vi "Interpret Driver Controls.vi"() -> ()   [LabVIEW 2018]
uses:
  <vilib>/Rock Robotics/WPI/DriverStation/WPI_DriverStationDerivedRobotMode.ctl
  Robot Global Data.vi
  SubSystems/Controllers/Driver Controller/Driver Controller Global.vi
  SubSystems/Drive Train/Drive Train Global.vi
  SubSystems/Lift/Lift Global.vi
  <vilib>/addons/control/pid/pid.llb/PID (DBL).vi
  SubSystems/Controllers/Manipulator Controlller/Manipulator Controller Global.vi
  SubSystems/HAB Climber/HAB Climber Global.vi
  SubSystems/Hatch Panel Intake/Hatch Panel Intake Global.vi
  SubSystems/Cargo Intake/Cargo Intake Global.vi
  <vilib>/addons/control/pid/NI_PID_pid.lvlib
panel:
  in  "Last Move Deadband":u32=500
  in  "Last Time Auto":u32=1171826
  in  "Camera Tracking":T1={"proportional gain (Kc)"=0.06, "integral time (Ti, min)"=0.0, "derivative time (Td, min)"=0.0}
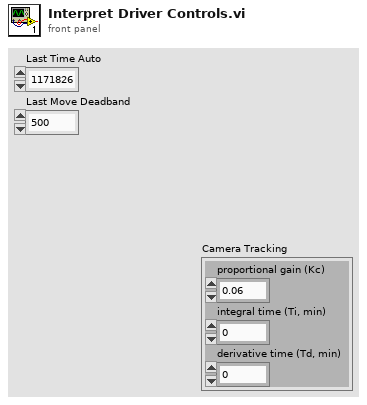
[diagram p1: front panel]
types:
  T1 = cluster{"proportional gain (Kc)":dbl, "integral time (Ti, min)":dbl, "derivative time (Td, min)":dbl}
  T2 = enum16{"Manual", "Hatch Panel Zone 1", "Hatch Panel Zone 2", "Hatch Panel Zone 3", "Cargo Zone 1", "Cargo Zone 2", "Cargo Zone 3", "Cargo Ship Zone"}
  T3 = cluster{"Rollover":dbl, "Yaw":dbl, "Cont Yaw":dbl}
  T4 = typedef "WPI_DriverStationDerivedRobotMode.ctl" = enum16{"Init", "Execute", "Stop"}
  T5 = enum16{"Hatch Panel Zone 1", "Hatch Panel Zone 2", "Hatch Panel Zone 3", "Cargo Zone 1", "Cargo Zone 2", "Cargo Zone 3", "Cargo Ship Zone"}
  T6 = cluster{"offsetAngle H":dbl, "offsetAngle V":dbl, "area":dbl, "skew":dbl, "validTarget":dbl, "latency":dbl}
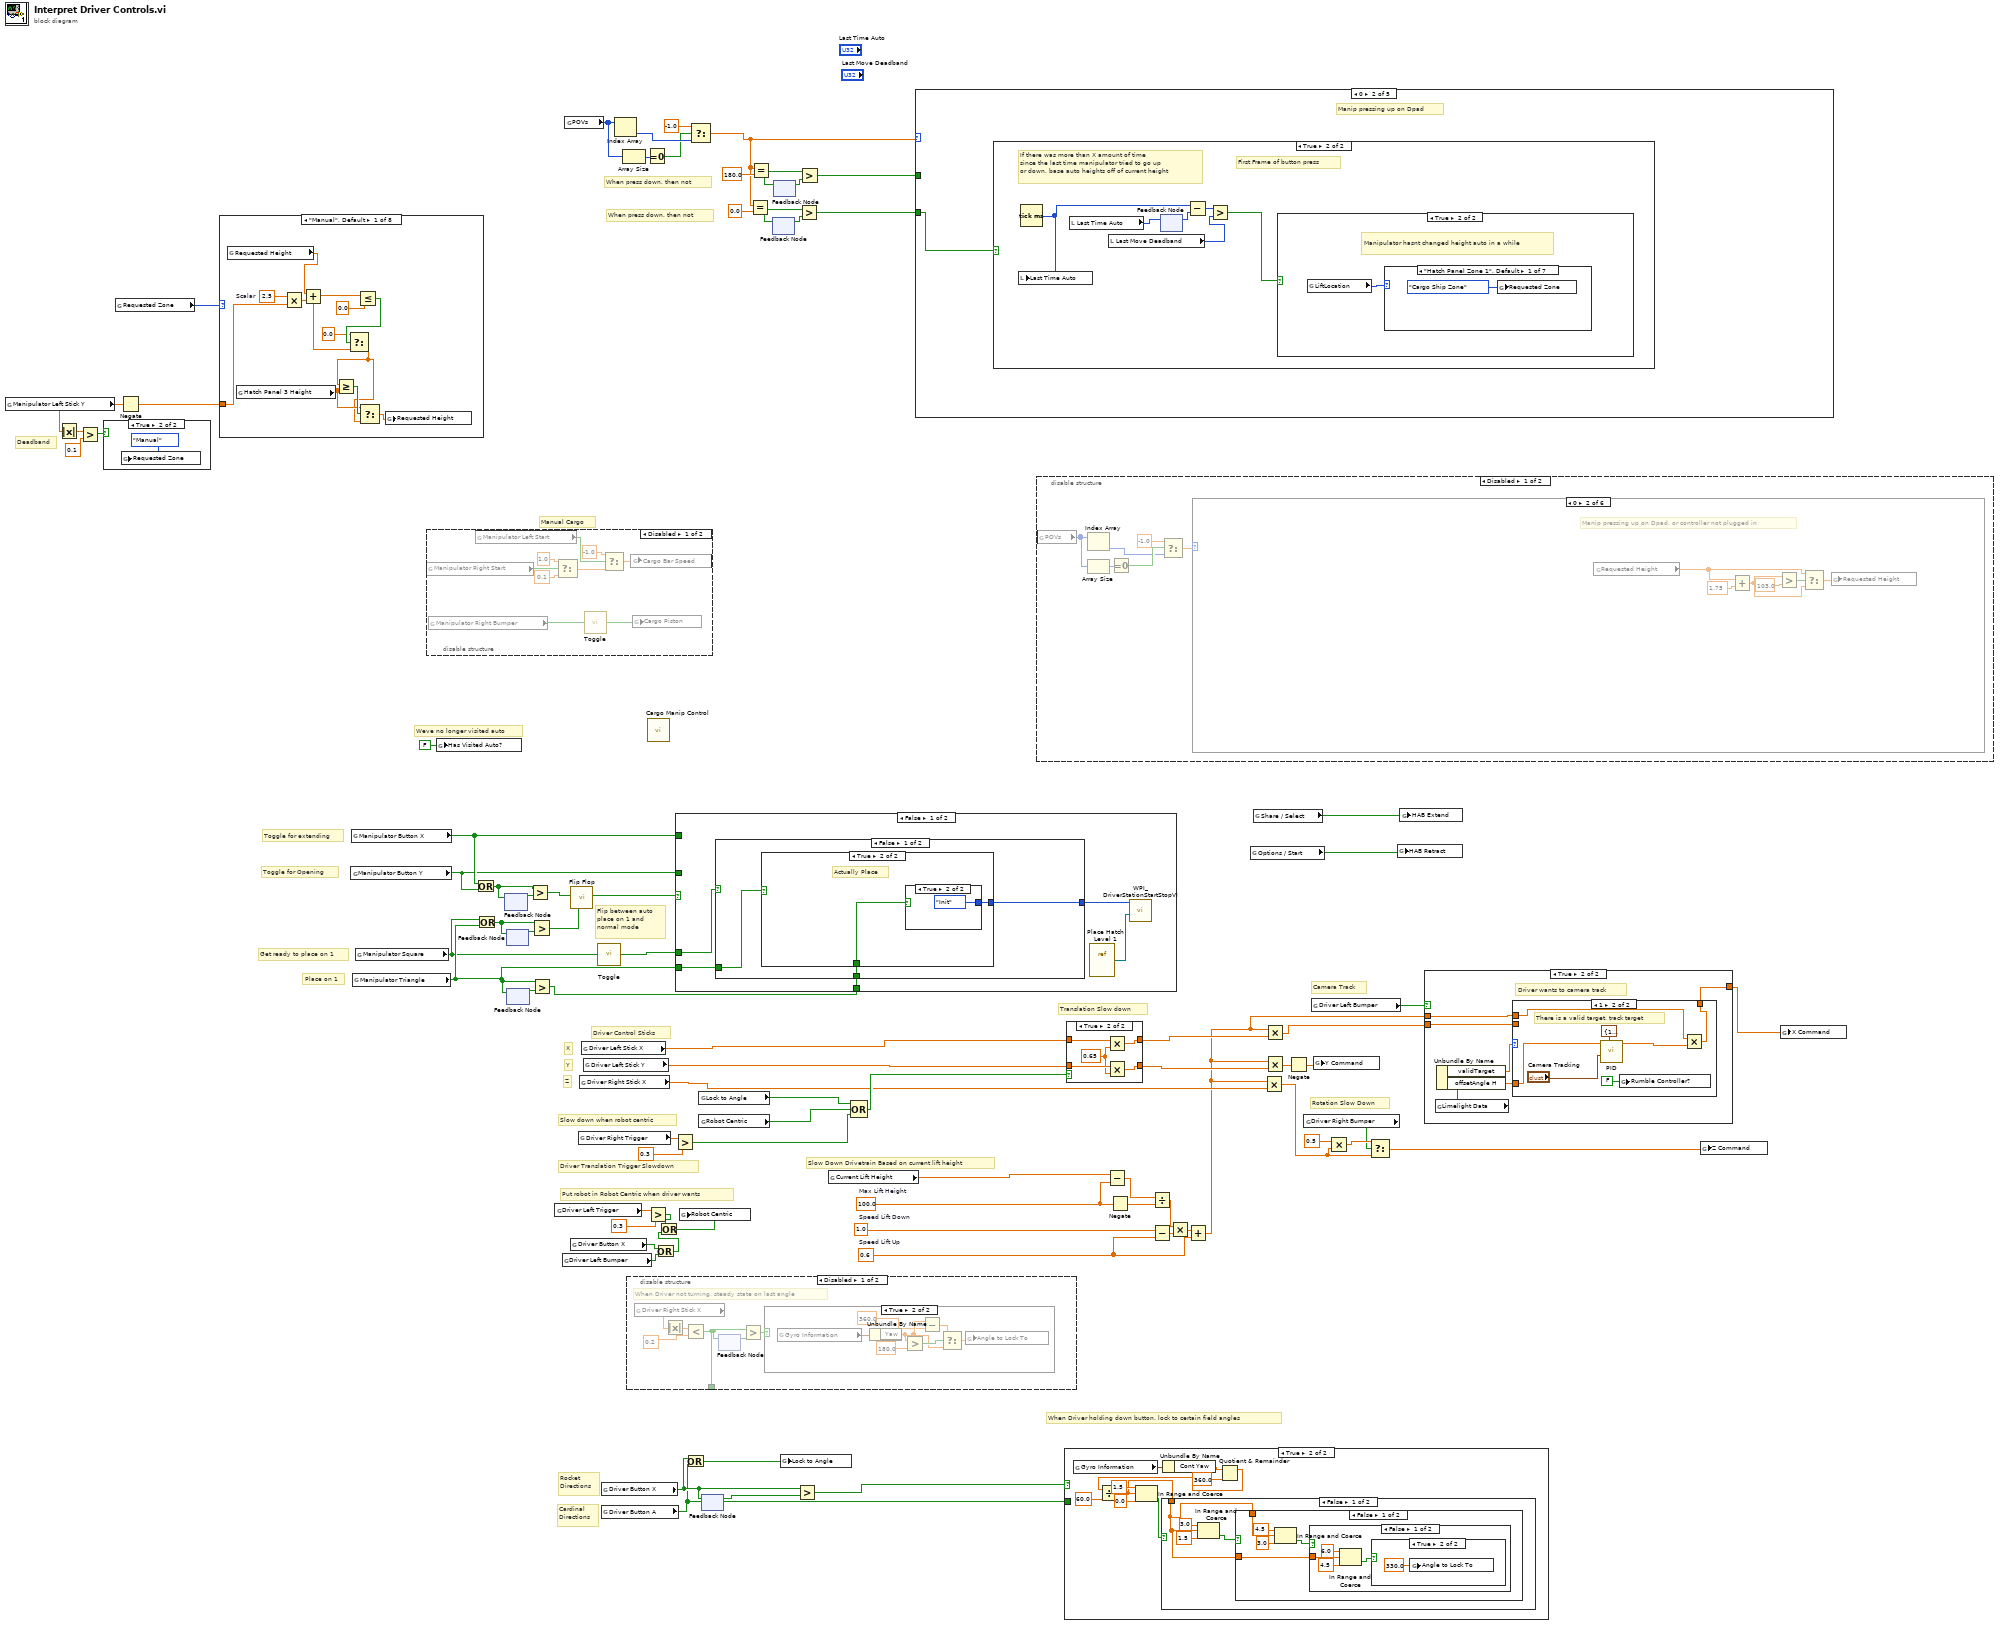
[diagram p0: block diagram]
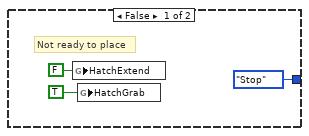
[diagram p2: hidden frame]
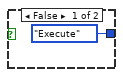
[diagram p3: hidden frame]
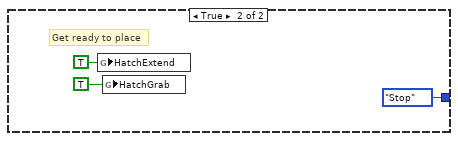
[diagram p4: hidden frame]
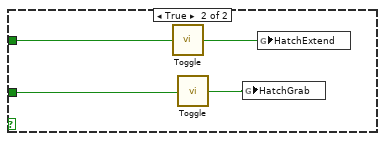
[diagram p5: hidden frame]
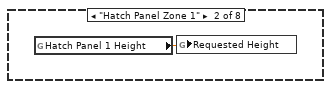
[diagram p7: hidden frame]
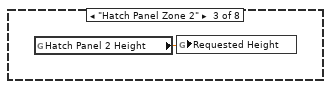
[diagram p8: hidden frame]
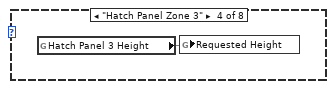
[diagram p9: hidden frame]
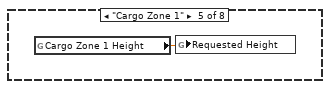
[diagram p10: hidden frame]
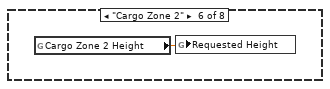
[diagram p11: hidden frame]
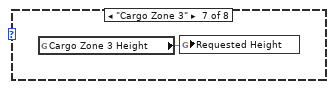
[diagram p12: hidden frame]
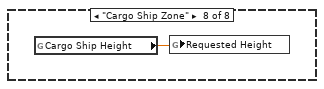
[diagram p13: hidden frame]
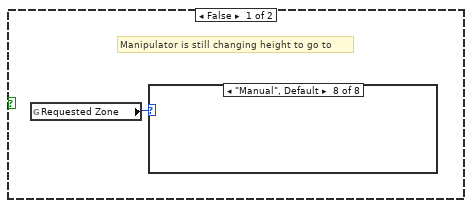
[diagram p16: hidden frame]
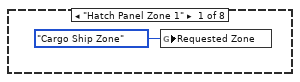
[diagram p17: hidden frame]
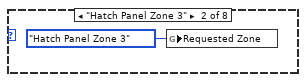
[diagram p18: hidden frame]
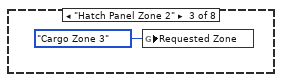
[diagram p19: hidden frame]
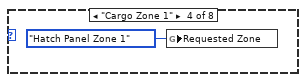
[diagram p20: hidden frame]
diagram:
  w60 = 0.6  # Speed Lift Up
  w64 = 1.0  # Speed Lift Down
  w58 = 100.0  # Max Lift Height
  # "Toggle for Opening"
  # "Toggle for extending"
  # "Place on 1"
  # "Get ready to place on 1"
  # "Flip between auto\nplace on 1 and \nnormal mode"
  # "When press down, then not"
  # "When press down, then not"
  # "Deadband"
  # "Manual Cargo"
  # "Weve no longer visited auto"
  # "Camera Track"
  # "Rotation Slow Down"
  # "Rocket\nDirections"
  # "Cardinal\nDirections"
  # "When Driver holding down button, lock to certain field angles"
  # "Slow Down Drivetrain Based on current lift height"
  # "Put robot in Robot Centric when driver wants"
  # "Slow down when robot centric"
  # "Driver Translation Trigger Slowdown"
  # "Translation Slow down"
  # "Z"
  # "Y"
  # "X"
  # "Driver Control Sticks"
  n1 = global read "Manipulator Controller Global.vi" "Manipulator Left Stick Y"() -> (w27:dbl)
  n2 = Absolute Value(x=w27) -> (abs(x)=w30:dbl)
  n3 = Greater?(x=w30, y=0.1) -> (0:w28:bool)
  n4 = case shown="True" w28 {
    frame False {
    }
    frame True {
      n5 = global write "Lift Global.vi" "Requested Zone"(T2."Manual" ("Requested Zone")) -> ()
    }
  }
  n6 = global read "Lift Global.vi" "Requested Zone"() -> (w31:T2)
  n7 = Negate(x=w27) -> (-x=w26:dbl)
  n8 = case shown="\"Manual\", Default" w31 {
    tunnel: w26 -> [w91 _ _ _ _ _ _ _]
    frame "Manual", Default {
      w90 = 2.5  # Scalar
      n9 = global read "Lift Global.vi" "Requested Height"() -> (w93:dbl)
      n10 = global read "Lift Global.vi" "Hatch Panel 3 Height"() -> (w84:dbl)
      n11 = Multiply(x=w90, y=w91) -> (x*y=w92:dbl)
      n12 = Add(x=w93, y=w92) -> (x+y=w86:dbl)
      n13 = Less Or Equal?(x=w86, y=0.0) -> (x <= y?=w88:bool)
      n14 = Select(t=0.0, s=w88, f=w86) -> (s? t:f=w83:dbl)
      n15 = Greater Or Equal?(x=w83, y=w84) -> (x >= y?=w85:bool)
      n16 = Select(t=w84, s=w85, f=w83) -> (s? t:f=w82:dbl)
      n17 = global write "Lift Global.vi" "Requested Height"(w82) -> ()
    }
    frame "Hatch Panel Zone 1" {
      n18 = global read "Lift Global.vi" "Hatch Panel 1 Height"() -> (w94:dbl)
      n19 = global write "Lift Global.vi" "Requested Height"(w94) -> ()
    }
    frame "Hatch Panel Zone 2" {
      n20 = global read "Lift Global.vi" "Hatch Panel 2 Height"() -> (w95:dbl)
      n21 = global write "Lift Global.vi" "Requested Height"(w95) -> ()
    }
    frame "Hatch Panel Zone 3" {
      n22 = global read "Lift Global.vi" "Hatch Panel 3 Height"() -> (w96:dbl)
      n23 = global write "Lift Global.vi" "Requested Height"(w96) -> ()
    }
    frame "Cargo Zone 1" {
      n24 = global read "Lift Global.vi" "Cargo Zone 1 Height"() -> (w97:dbl)
      n25 = global write "Lift Global.vi" "Requested Height"(w97) -> ()
    }
    frame "Cargo Zone 2" {
      n26 = global read "Lift Global.vi" "Cargo Zone 2 Height"() -> (w98:dbl)
      n27 = global write "Lift Global.vi" "Requested Height"(w98) -> ()
    }
    frame "Cargo Zone 3" {
      n28 = global read "Lift Global.vi" "Cargo Zone 3 Height"() -> (w99:dbl)
      n29 = global write "Lift Global.vi" "Requested Height"(w99) -> ()
    }
    frame "Cargo Ship Zone" {
      n30 = global read "Lift Global.vi" "Cargo Ship Height"() -> (w100:dbl)
      n31 = global write "Lift Global.vi" "Requested Height"(w100) -> ()
    }
  }
  n32 = global read "Manipulator Controller Global.vi" "Manipulator Button Y"() -> (w13:bool)
  n33 = global read "Manipulator Controller Global.vi" "Manipulator Button X"() -> (w14:bool)
  n34 = global read "Manipulator Controller Global.vi" "Manipulator Triangle"() -> (w3:bool)
  n35 = global read "Manipulator Controller Global.vi" "Manipulator Square"() -> (w2:bool)
  n36 = disable-structure shown="Disabled" {
    frame Disabled {
      n37 = global read "Manipulator Controller Global.vi" "Manipulator Right Start"() -> (w106:bool)
      n38 = global read "Manipulator Controller Global.vi" "Manipulator Right Bumper"() -> (w109:bool)
      n39 = global read "Manipulator Controller Global.vi" "Manipulator Left Start"() -> (w105:bool)
      n40 = Select(t=1.0, s=w106, f=0.1) -> (s? t:f=w104:dbl)
      n41 = call "Toggle.vi"("Input"=w109) -> ("Output"=w108:bool)
      n42 = Select(t=-1.0, s=w105, f=w104) -> (s? t:f=w107:dbl)
      n43 = global write "Cargo Intake Global.vi" "Cargo Bar Speed"(w107) -> ()
      n44 = global write "Cargo Intake Global.vi" "Cargo Piston"(w108) -> ()
    }
    frame Enabled {
    }
  }
  n45 = global write "Robot Global Data.vi" "Has Visited Auto?"(FALSE ("Has Visited Auto?")) -> ()
  n46 = Or(x=w14, y=w13) -> (x .or. y?=w11:bool)
  n47 = Or(x=w2, y=w3) -> (x .or. y?=w8:bool)
  n48 = feedback-in #1(w11) -> ()
  n49 = feedback #1() -> (w12:bool)  [unwired: 1 in]
  n50 = feedback #2() -> (w9:bool)  [unwired: 1 in]
  n51 = feedback-in #2(w8) -> ()
  n52 = feedback #3() -> (w5:bool)  [unwired: 1 in]
  n53 = feedback-in #3(w3) -> ()
  n54 = Greater?(x=w11, y=w12) -> (0:w10:bool)
  n55 = Greater?(x=w8, y=w9) -> (0:w7:bool)
  n56 = Greater?(x=w3, y=w5) -> (0:w4:bool)
  n57 = global read "Driver Controller Global.vi" "Driver Left Trigger"() -> (w77:dbl)
  n58 = global read "Driver Controller Global.vi" "Driver Left Bumper"() -> (w43:bool)
  n59 = global read "Manipulator Controller Global.vi" "POVs"() -> (w35:i16[])
  n60 = call "Flip Flop.vi"("Line 2"=w7, "Line 1"=w10) -> ("Switch"=w6:bool)  [unwired: 9 in]
  n61 = global read "Driver Controller Global.vi" "Driver Button X"() -> (w44:bool)
  n62 = global read "Driver Controller Global.vi" "Driver Right Trigger"() -> (w80:dbl)
  n63 = global read "Driver Controller Global.vi" "Driver Right Stick X"() -> (w36:dbl)
  n64 = global read "Driver Controller Global.vi" "Driver Left Stick X"() -> (w37:dbl)
  n65 = global read "Driver Controller Global.vi" "Driver Left Stick Y"() -> (w67:dbl)
  n66 = call "Toggle.vi"("Input"=w2) -> ("Output"=w1:bool)
  n67 = global read "Driver Controller Global.vi" "Driver Button X"() -> (w56:bool)
  n68 = global read "Driver Controller Global.vi" "Driver Button A"() -> (w54:bool)
  n69 = Index Array(array=w35) -> (element=w32:i16)  [unwired: 1 in]
  n70 = Array Size(array=w35) -> (size(s)=w34:i32)
  n71 = disable-structure shown="Disabled" {
    disable-tunnel: [w110 _] -> _
    frame Disabled {
      # "When Driver not turning, steady state on last angle"
      n72 = global read "Driver Controller Global.vi" "Driver Right Stick X"() -> (w111:dbl)
      n73 = Absolute Value(x=w111) -> (abs(x)=w115:dbl)
      n74 = Less?(x=w115, y=0.2) -> (x < y?=w110:bool)
      n75 = feedback #4() -> (w113:bool)  [unwired: 1 in]
      n76 = feedback-in #4(w110) -> ()
      n77 = Greater?(x=w110, y=w113) -> (0:w112:bool)
      n78 = case shown="True" w112 {
        frame False {
        }
        frame True {
          n79 = global read "Drive Train Global.vi" "Gyro Information"() -> (w122:T3)
          n80 = Unbundle By Name(w122) -> ("Yaw"=w119:dbl)
          n81 = Greater?(x=w119, y=180.0) -> (0:w120:bool)
          n82 = Subtract(x=w119, y=360.0) -> (x-y=w117:dbl)
          n83 = Select(t=w117, s=w120, f=w119) -> (s? t:f=w116:dbl)
          n84 = global write "Drive Train Global.vi" "Angle to Lock To"(w116) -> ()
        }
      }
    }
    frame Enabled {
    }
  }
  n85 = Equal To 0?(x=w34) -> (x = 0?=w25:bool)
  n86 = call "Cargo Manip Control.vi"() -> ()  [unwired: 12 in]
  n87 = Greater?(x=w77, y=0.3) -> (0:w52:bool)
  n88 = Or(x=w44, y=w43) -> (x .or. y?=w45:bool)
  n89 = Or(x=w52, y=w45) -> (x .or. y?=w50:bool)
  n90 = Greater?(x=w80, y=0.3) -> (0:w72:bool)
  n91 = case shown="False" w6 {
    tunnel: w13 -> [_ w144]
    tunnel: w14 -> [_ w142]
    tunnel: w1 -> [w127 _]
    tunnel: w4 -> [w124 _]
    tunnel: w3 -> [w123 _]
    frame False {
      n92 = case shown="False" w127 {
        tunnel: [w130 WPI_DriverStationDerivedRobotMode."Stop" ("Call Context")] -> w125
        tunnel: w124 -> [w129 _]
        tunnel: w123 -> [w128 _]
        frame False {
          n93 = case shown="True" w128 {
            tunnel: [WPI_DriverStationDerivedRobotMode."Stop" ("Call Context") w135] -> w130
            tunnel: w129 -> [_ w134]
            frame False {
              # "Not ready to place"
              n94 = global write "Hatch Panel Intake Global.vi" "HatchExtend"(FALSE ("HatchExtend")) -> ()
              n95 = global write "Hatch Panel Intake Global.vi" "HatchGrab"(TRUE ("HatchExtend")) -> ()
            }
            frame True {
              # "Actually Place"
              n96 = case shown="True" w134 {
                tunnel: [WPI_DriverStationDerivedRobotMode."Execute" ("Call Context") WPI_DriverStationDerivedRobotMode."Init" ("Call Context")] -> w135
                frame False {
                }
                frame True {
                }
              }
            }
          }
        }
        frame True {
          # "Get ready to place"
          n97 = global write "Hatch Panel Intake Global.vi" "HatchExtend"(TRUE ("HatchExtend")) -> ()
          n98 = global write "Hatch Panel Intake Global.vi" "HatchGrab"(TRUE ("HatchExtend")) -> ()
        }
      }
      n99 = vi-ref "Place Hatch Level 1.vi"() -> (w126:refnum<vi>)
      n100 = call <vilib>:"WPI_DriverStationStartStopVI.vi"("VI in"=w126, "Call Context"=w125) -> ()  [unwired: 10 in]
    }
    frame True {
      n101 = call "Toggle.vi"("Input"=w142) -> ("Output"=w143:bool)
      n102 = call "Toggle.vi"("Input"=w144) -> ("Output"=w141:bool)
      n103 = global write "Hatch Panel Intake Global.vi" "HatchGrab"(w141) -> ()
      n104 = global write "Hatch Panel Intake Global.vi" "HatchExtend"(w143) -> ()
    }
  }
  n105 = global write "Drive Train Global.vi" "Robot Centric"(w50) -> ()
  n106 = Or(x=w56, y=w54) -> (x .or. y?=w53:bool)
  n107 = Select(t=-1.0, s=w25, f=w32) -> (s? t:f=w17:dbl)
  n108 = global read "Drive Train Global.vi" "Lock to Angle"() -> (w51:bool)
  n109 = global read "Drive Train Global.vi" "Robot Centric"() -> (w71:bool)
  n110 = feedback #5() -> (w57:bool)  [unwired: 1 in]
  n111 = feedback-in #5(w56) -> ()
  n112 = Equal?(x=w17, y=0.0) -> (x = y?=w20:bool)
  n113 = Equal?(x=w17, y=180.0) -> (x = y?=w22:bool)
  n114 = feedback #6() -> (w19:bool)  [unwired: 1 in]
  n115 = feedback-in #6(w20) -> ()
  n116 = feedback-in #7(w22) -> ()
  n117 = feedback #7() -> (w23:bool)  [unwired: 1 in]
  n118 = global write "Drive Train Global.vi" "Lock to Angle"(w53) -> ()
  n119 = Greater?(x=w56, y=w57) -> (0:w55:bool)
  n120 = Greater?(x=w20, y=w19) -> (0:w16:bool)
  n121 = Greater?(x=w22, y=w23) -> (0:w21:bool)
  n122 = global read "Lift Global.vi" "Current Lift Height"() -> (w66:dbl)
  n123 = Compound Arithmetic op=OR(w51, w71, w72) -> (w70:bool)
  n124 = case shown="0" w17 {
    tunnel: w21 -> [_ _ w168 _ _]
    tunnel: w16 -> [_ w145 _ _ _]
    frame -1, Default {
      # "Nothing on the D-Pad is pressed!"
    }
    frame 0 {
      # "Manip pressing up on Dpad"
      n125 = case shown="True" w145 {
        frame False {
          # "Still pressing button, do nothing"
        }
        frame True {
          # "First Frame of button press"
          # "If there was more than X amount of time\nsince the last time manipulator tried to go up\nor down, base auto heights off of current height"
          n126 = Tick Count (ms)() -> (millisecond timer value=w148:u32)
          n127 = local write "Last Time Auto"(w148) -> ()
          n128 = local read "Last Time Auto"() -> (w147:u32)
          n129 = local read "Last Move Deadband"() -> (w149:u32)
          n130 = feedback #8() -> (w146:u32)  [unwired: 1 in]
          n131 = feedback-in #8(w147) -> ()
          n132 = Subtract(x=w148, y=w146) -> (x-y=w151:u32)
          n133 = Greater?(x=w151, y=w149) -> (0:w150:bool)
          n134 = case shown="True" w150 {
            frame False {
              # "Manipulator is still changing height to go to"
              n135 = global read "Lift Global.vi" "Requested Zone"() -> (w152:T2)
              n136 = case shown="\"Manual\", Default" w152 {
                frame "Hatch Panel Zone 1" {
                  n137 = global write "Lift Global.vi" "Requested Zone"(T2."Cargo Ship Zone" ("Requested Zone")) -> ()
                }
                frame "Hatch Panel Zone 3" {
                  n138 = global write "Lift Global.vi" "Requested Zone"(T2."Hatch Panel Zone 3" ("Requested Zone")) -> ()
                }
                frame "Hatch Panel Zone 2" {
                  n139 = global write "Lift Global.vi" "Requested Zone"(T2."Cargo Zone 3" ("Requested Zone")) -> ()
                }
                frame "Cargo Zone 1" {
                  n140 = global write "Lift Global.vi" "Requested Zone"(T2."Hatch Panel Zone 1" ("Requested Zone")) -> ()
                }
                frame "Cargo Zone 2" {
                  n141 = global write "Lift Global.vi" "Requested Zone"(T2."Hatch Panel Zone 2" ("Requested Zone")) -> ()
                }
                frame "Cargo Zone 3" {
                  n142 = global write "Lift Global.vi" "Requested Zone"(T2."Hatch Panel Zone 3" ("Requested Zone")) -> ()
                }
                frame "Cargo Ship Zone" {
                  n143 = global write "Lift Global.vi" "Requested Zone"(T2."Cargo Zone 2" ("Requested Zone")) -> ()
                }
                frame "Manual", Default {
                }
              }
            }
            frame True {
              # "Manipulator hasnt changed height auto in a while"
              n144 = global read "Lift Global.vi" "LiftLocation"() -> (w160:T5)
              n145 = case shown="\"Hatch Panel Zone 1\", Default" w160 {
                frame "Hatch Panel Zone 1", Default {
                  n146 = global write "Lift Global.vi" "Requested Zone"(T2."Cargo Ship Zone" ("Requested Zone")) -> ()
                }
                frame "Hatch Panel Zone 3" {
                  n147 = global write "Lift Global.vi" "Requested Zone"(T2."Hatch Panel Zone 3" ("Requested Zone")) -> ()
                }
                frame "Hatch Panel Zone 2" {
                  n148 = global write "Lift Global.vi" "Requested Zone"(T2."Cargo Zone 3" ("Requested Zone")) -> ()
                }
                frame "Cargo Zone 1" {
                  n149 = global write "Lift Global.vi" "Requested Zone"(T2."Hatch Panel Zone 1" ("Requested Zone")) -> ()
                }
                frame "Cargo Zone 2" {
                  n150 = global write "Lift Global.vi" "Requested Zone"(T2."Hatch Panel Zone 2" ("Requested Zone")) -> ()
                }
                frame "Cargo Zone 3" {
                  n151 = global write "Lift Global.vi" "Requested Zone"(T2."Hatch Panel Zone 3" ("Requested Zone")) -> ()
                }
                frame "Cargo Ship Zone" {
                  n152 = global write "Lift Global.vi" "Requested Zone"(T2."Cargo Zone 2" ("Requested Zone")) -> ()
                }
              }
            }
          }
        }
      }
    }
    frame 180 {
      # "Manip pressing down on Dpad"
      n153 = case shown="True" w168 {
        frame False {
          # "Still pressing button, do nothing"
        }
        frame True {
          # "First frame of button press"
          # "If there was more than X amount of time\nsince the last time manipulator tried to go up\nor down, base auto heights off of current height"
          n154 = Tick Count (ms)() -> (millisecond timer value=w173:u32)
          n155 = local write "Last Time Auto"(w173) -> ()
          n156 = local read "Last Time Auto"() -> (w170:u32)
          n157 = local read "Last Move Deadband"() -> (w172:u32)
          n158 = feedback #9() -> (w169:u32)  [unwired: 1 in]
          n159 = feedback-in #9(w170) -> ()
          n160 = Subtract(x=w173, y=w169) -> (x-y=w174:u32)
          n161 = Greater?(x=w174, y=w172) -> (0:w171:bool)
          n162 = case shown="False" w171 {
            frame False {
              # "Manipulator is still changing height to go to"
              n163 = global read "Lift Global.vi" "Requested Zone"() -> (w175:T2)
              n164 = case shown="\"Cargo Ship Zone\"" w175 {
                frame "Hatch Panel Zone 1" {
                  n165 = global write "Lift Global.vi" "Requested Zone"(T2."Cargo Zone 1" ("Requested Zone")) -> ()
                }
                frame "Hatch Panel Zone 3" {
                  n166 = global write "Lift Global.vi" "Requested Zone"(T2."Cargo Zone 3" ("Requested Zone")) -> ()
                }
                frame "Hatch Panel Zone 2" {
                  n167 = global write "Lift Global.vi" "Requested Zone"(T2."Cargo Zone 2" ("Requested Zone")) -> ()
                }
                frame "Cargo Zone 1" {
                  n168 = global write "Lift Global.vi" "Requested Zone"(T2."Cargo Zone 1" ("Requested Zone")) -> ()
                }
                frame "Cargo Zone 2" {
                  n169 = global write "Lift Global.vi" "Requested Zone"(T2."Cargo Ship Zone" ("Requested Zone")) -> ()
                }
                frame "Cargo Zone 3" {
                  n170 = global write "Lift Global.vi" "Requested Zone"(T2."Hatch Panel Zone 2" ("Requested Zone")) -> ()
                }
                frame "Cargo Ship Zone" {
                  n171 = global write "Lift Global.vi" "Requested Zone"(T2."Hatch Panel Zone 1" ("Requested Zone")) -> ()
                }
                frame "Manual", Default {
                }
              }
            }
            frame True {
              # "Manipulator hasnt changed height auto in a while"
              n172 = global read "Lift Global.vi" "LiftLocation"() -> (w183:T5)
              n173 = case shown="\"Hatch Panel Zone 1\", Default" w183 {
                frame "Hatch Panel Zone 1", Default {
                  n174 = global write "Lift Global.vi" "Requested Zone"(T2."Cargo Zone 1" ("Requested Zone")) -> ()
                }
                frame "Hatch Panel Zone 3" {
                  n175 = global write "Lift Global.vi" "Requested Zone"(T2."Cargo Zone 3" ("Requested Zone")) -> ()
                }
                frame "Hatch Panel Zone 2" {
                  n176 = global write "Lift Global.vi" "Requested Zone"(T2."Cargo Zone 2" ("Requested Zone")) -> ()
                }
                frame "Cargo Zone 1" {
                  n177 = global write "Lift Global.vi" "Requested Zone"(T2."Cargo Zone 1" ("Requested Zone")) -> ()
                }
                frame "Cargo Zone 2" {
                  n178 = global write "Lift Global.vi" "Requested Zone"(T2."Cargo Ship Zone" ("Requested Zone")) -> ()
                }
                frame "Cargo Zone 3" {
                  n179 = global write "Lift Global.vi" "Requested Zone"(T2."Hatch Panel Zone 2" ("Requested Zone")) -> ()
                }
                frame "Cargo Ship Zone" {
                  n180 = global write "Lift Global.vi" "Requested Zone"(T2."Hatch Panel Zone 1" ("Requested Zone")) -> ()
                }
              }
            }
          }
        }
      }
    }
    frame 90 {
      # "Go to Cargo in Cargo Ship Height"
      # "Right on D-Pad"
      n181 = global write "Lift Global.vi" "Requested Zone"(T2."Cargo Ship Zone" ("Requested Zone")) -> ()
    }
    frame 270 {
      # "Go to Hatch Level 1 Height"
      # "Left on D-Pad"
      n182 = global write "Lift Global.vi" "Requested Zone"(T2."Hatch Panel Zone 1" ("Requested Zone")) -> ()
    }
  }
  n183 = disable-structure shown="Disabled" {
    frame Disabled {
      n184 = global read "Manipulator Controller Global.vi" "POVs"() -> (w198:i16[])
      n185 = Index Array(array=w198) -> (element=w193:i16)  [unwired: 1 in]
      n186 = Array Size(array=w198) -> (size(s)=w197:i32)
      n187 = Equal To 0?(x=w197) -> (x = 0?=w195:bool)
      n188 = Select(t=-1.0, s=w195, f=w193) -> (s? t:f=w196:dbl)
      n189 = case shown="0" w196 {
        frame -1 {
          # "If the value changed (manip pressed button)\nchange set lift height to match"
          # "When button goes from\nnot pressed to pressed"
          n190 = global read "Manipulator Controller Global.vi" "Manipulator Square"() -> (w204:bool)
          n191 = feedback #10() -> (w205:bool)  [unwired: 1 in]
          n192 = feedback-in #10(w204) -> ()
          n193 = Greater?(x=w204, y=w205) -> (0:w201:bool)
          n194 = feedback #11() -> (w199:dbl)  [unwired: 1 in]
          n195 = feedback #12() -> (w203:dbl)  [unwired: 1 in]
          n196 = case shown="False" w201 {
            tunnel: [w215 w230] -> w200
            tunnel: w203 -> [w216 w229]
            frame False {
              # "When button goes from\nnot pressed to pressed"
              n197 = global read "Manipulator Controller Global.vi" "Manipulator Triangle"() -> (w218:bool)
              n198 = feedback #13() -> (w217:bool)  [unwired: 1 in]
              n199 = feedback-in #13(w218) -> ()
              n200 = Greater?(x=w218, y=w217) -> (0:w214:bool)
              n201 = case shown="True" w214 {
                tunnel: w216 -> [w219 w221]
                tunnel: [w219 w223] -> w215
                frame False {
                }
                frame True {
                  # "If counter smaller than 5\nadd 1"
                  n202 = Less?(x=w221, y=5.0) -> (x < y?=w220:bool)
                  n203 = case shown="True" w220 {
                    tunnel: [w224 w226] -> w223
                    tunnel: w221 -> [w224 w225]
                    frame False {
                    }
                    frame True {
                      n204 = Increment(x=w225) -> (x+1=w226:dbl)
                    }
                  }
                }
              }
            }
            frame True {
              # "If counter bigger than 0\nsubtract 1"
              n205 = Greater?(x=w229, y=0.0) -> (0:w228:bool)
              n206 = case shown="False" w228 {
                tunnel: [0.0 ("y") w233] -> w230
                tunnel: w229 -> [_ w232]
                frame False {
                }
                frame True {
                  n207 = Decrement(x=w232) -> (x-1=w233:dbl)
                }
              }
            }
          }
          n208 = feedback-in #11(w200) -> ()
          n209 = Not Equal?(x=w200, y=w199) -> (x != y?=w202:bool)
          n210 = case shown="True" w202 {
            tunnel: w200 -> [_ w206]
            frame False {
              # "Manipulator didnt request change"
            }
            frame True {
              # "Set height request to new value"
              n211 = case shown="0, Default" w206 {
                tunnel: [w208 w209 w210 w211 w212 w213] -> w207
                frame 0, Default {
                  n212 = global read "Lift Global.vi" "Cargo Zone 1 Height"() -> (w208:dbl)
                }
                frame 1 {
                  n213 = global read "Lift Global.vi" "Hatch Panel 1 Height"() -> (w209:dbl)
                }
                frame 2 {
                  n214 = global read "Lift Global.vi" "Cargo Zone 2 Height"() -> (w210:dbl)
                }
                frame 3 {
                  n215 = global read "Lift Global.vi" "Hatch Panel 2 Height"() -> (w211:dbl)
                }
                frame 4 {
                  n216 = global read "Lift Global.vi" "Cargo Zone 3 Height"() -> (w212:dbl)
                }
                frame 5 {
                  n217 = global read "Lift Global.vi" "Hatch Panel 3 Height"() -> (w213:dbl)
                }
              }
              n218 = global write "Lift Global.vi" "Requested Height"(w207) -> ()
            }
          }
          n219 = global write "Lift Global.vi" "Lift Auto Position"(w200) -> ()
          n220 = feedback-in #12(w200) -> ()
        }
        frame 0 {
          # "Manip pressing up on Dpad, or controller not plugged in"
          n221 = global read "Lift Global.vi" "Requested Height"() -> (w235:dbl)
          n222 = Add(x=w235, y=1.75) -> (x+y=w234:dbl)
          n223 = Greater?(x=w234, y=103.0) -> (0:w236:bool)
          n224 = Select(t=w235, s=w236, f=w234) -> (s? t:f=w237:dbl)
          n225 = global write "Lift Global.vi" "Requested Height"(w237) -> ()
        }
        frame 180 {
          # "Manip pressing down on Dpad"
          n226 = global read "Lift Global.vi" "Requested Height"() -> (w240:dbl)
          n227 = Add(x=w240, y=-1.0) -> (x+y=w242:dbl)
          n228 = Less?(x=w242, y=0.0) -> (x < y?=w243:bool)
          n229 = Select(t=w240, s=w243, f=w242) -> (s? t:f=w241:dbl)
          n230 = global write "Lift Global.vi" "Requested Height"(w241) -> ()
        }
        frame 90 {
          # "Go to Cargo in Cargo Ship Height"
          # "Right on D-Pad"
          n231 = global read "Lift Global.vi" "Cargo Ship Height"() -> (w246:dbl)
          n232 = global write "Lift Global.vi" "Requested Height"(w246) -> ()
        }
        frame 270 {
          # "Go to Hatch Level 1 Height"
          # "Left on D-Pad"
          n233 = global read "Lift Global.vi" "Hatch Panel 1 Height"() -> (w247:dbl)
          n234 = global write "Lift Global.vi" "Requested Height"(w247) -> ()
        }
        frame -100, Default {
        }
      }
    }
    frame Enabled {
    }
  }
  n235 = case shown="True" w55 {
    tunnel: w54 -> [w249 _]
    frame False {
      n236 = feedback #14() -> (w250:bool)  [unwired: 1 in]
      n237 = feedback-in #14(w249) -> ()
      n238 = Greater?(x=w249, y=w250) -> (0:w248:bool)
      n239 = case shown="True" w248 {
        frame False {
        }
        frame True {
          n240 = global read "Drive Train Global.vi" "Gyro Information"() -> (w257:T3)
          n241 = Unbundle By Name(w257) -> ("Yaw"=w254:dbl)
          n242 = Add(x=w254, y=180.0) -> (x+y=w253:dbl)
          n243 = Divide(x=w253, y=90.0) -> (x/y=w255:dbl)
          n244 = Round To Nearest(number=w255) -> (nearest integer value=w251:dbl)
          n245 = case shown="1" w251 {
            frame 0, Default {
              n246 = global write "Drive Train Global.vi" "Angle to Lock To"(180.0 ("Angle to Lock To")) -> ()
            }
            frame 1 {
              n247 = global write "Drive Train Global.vi" "Angle to Lock To"(270.0 ("Angle to Lock To")) -> ()
            }
            frame 2 {
              n248 = global write "Drive Train Global.vi" "Angle to Lock To"(0.0 ("Angle to Lock To")) -> ()
            }
            frame 3 {
              n249 = global write "Drive Train Global.vi" "Angle to Lock To"(90.0 ("Angle to Lock To")) -> ()
            }
            frame 4 {
              n250 = global write "Drive Train Global.vi" "Angle to Lock To"(180.0 ("Angle to Lock To")) -> ()
            }
          }
        }
      }
    }
    frame True {
      n251 = global read "Drive Train Global.vi" "Gyro Information"() -> (w271:T3)
      n252 = Unbundle By Name(w271) -> ("Cont Yaw"=w269:dbl)
      n253 = Quotient & Remainder(x=w269, y=360.0) -> (x-y*floor(x/y)=w267:dbl)  [unwired: 1 out]
      n254 = Divide(x=w267, y=60.0) -> (x/y=w263:dbl)
      n255 = In Range and Coerce(upper limit=1.5, x=w263, lower limit=0.0) -> (In Range?=w264:bool)  [unwired: 1 out]
      n256 = case shown="False" w264 {
        tunnel: w263 -> [w272 _]
        frame False {
          n257 = In Range and Coerce(upper limit=3.0, x=w272, lower limit=1.5) -> (In Range?=w273:bool)  [unwired: 1 out]
          n258 = case shown="False" w273 {
            tunnel: w272 -> [w278 _]
            tunnel: w272 -> [w276 _]
            frame False {
              n259 = In Range and Coerce(upper limit=4.5, x=w278, lower limit=3.0) -> (In Range?=w277:bool)  [unwired: 1 out]
              n260 = case shown="False" w277 {
                tunnel: w276 -> [w282 _]
                frame False {
                  n261 = In Range and Coerce(upper limit=6.0, x=w282, lower limit=4.5) -> (In Range?=w281:bool)  [unwired: 1 out]
                  n262 = case shown="True" w281 {
                    frame False {
                    }
                    frame True {
                      n263 = global write "Drive Train Global.vi" "Angle to Lock To"(330.0 ("Angle to Lock To")) -> ()
                    }
                  }
                }
                frame True {
                  n264 = global write "Drive Train Global.vi" "Angle to Lock To"(210.0 ("Angle to Lock To")) -> ()
                }
              }
            }
            frame True {
              n265 = global write "Drive Train Global.vi" "Angle to Lock To"(150.0 ("Angle to Lock To")) -> ()
            }
          }
        }
        frame True {
          n266 = global write "Drive Train Global.vi" "Angle to Lock To"(30.0 ("Angle to Lock To")) -> ()
        }
      }
    }
  }
  n267 = case shown="True" w70 {
    tunnel: w67 -> [w290 w295]
    tunnel: [w290 w294] -> w69
    tunnel: [w289 w293] -> w68
    tunnel: w37 -> [w289 w292]
    frame False {
    }
    frame True {
      w291 = 0.65 ("Y Slower")
      n268 = Multiply(x=w292, y=w291) -> (x*y=w293:dbl)
      n269 = Multiply(x=w295, y=w291) -> (x*y=w294:dbl)
    }
  }
  n270 = Subtract(x=w66, y=w58) -> (x-y=w65:dbl)
  n271 = Negate(x=w58) -> (-x=w59:dbl)
  n272 = Divide(x=w65, y=w59) -> (x/y=w63:dbl)
  n273 = Subtract(x=w64, y=w60) -> (x-y=w62:dbl)
  n274 = Multiply(x=w63, y=w62) -> (x*y=w61:dbl)
  n275 = Add(x=w61, y=w60) -> (x+y=w15:dbl)
  n276 = global read "Manipulator Controller Global.vi" "Options / Start"() -> (w41:bool)
  n277 = global read "Manipulator Controller Global.vi" "Share / Select"() -> (w42:bool)
  n278 = Multiply(x=w15, y=w36) -> (x*y=w76:dbl)
  n279 = Multiply(x=w15, y=w68) -> (x*y=w47:dbl)
  n280 = Multiply(x=w15, y=w69) -> (x*y=w40:dbl)
  n281 = Negate(x=w40) -> (-x=w39:dbl)
  n282 = global read "Driver Controller Global.vi" "Driver Right Bumper"() -> (w73:bool)
  n283 = global read "Driver Controller Global.vi" "Driver Left Bumper"() -> (w49:bool)
  n284 = global write "Drive Train Global.vi" "Y Command"(w39) -> ()
  n285 = Multiply(x=0.5, y=w76) -> (x*y=w75:dbl)
  n286 = Select(t=w75, s=w73, f=w76) -> (s? t:f=w48:dbl)
  n287 = global write "HAB Climber Global.vi" "HAB Retract"(w41) -> ()
  n288 = global write "HAB Climber Global.vi" "HAB Extend"(w42) -> ()
  n289 = case shown="True" w49 {
    tunnel: w47 -> [w297 w301]
    tunnel: [w297 w299] -> w46
    tunnel: w15 -> [_ w298]
    frame False {
      # "Driver not attepting to camera track, be normal"
      n290 = global write "Driver Controller Global.vi" "Rumble Controller?"(FALSE ("Rumble Controller?")) -> ()
    }
    frame True {
      # "Driver wants to camera track"
      n291 = global read "Robot Global Data.vi" "Limelight Data"() -> (w303:T6)
      n292 = Unbundle By Name(w303) -> ("validTarget"=w302:dbl, "offsetAngle H"=w300:dbl)
      n293 = case shown="1" w302 {
        tunnel: w301 -> [w304 _]
        tunnel: w300 -> [_ w309]
        tunnel: [w304 w308] -> w299
        tunnel: w298 -> [_ w306]
        frame 0, Default {
          # "No Valid Target, keep using driver controls\nand rumble controller so knows not tracking"
          n294 = global write "Driver Controller Global.vi" "Rumble Controller?"(TRUE ("Rumble Controller?")) -> ()
        }
        frame 1 {
          # "There is a valid target, track target"
          n295 = call-poly <vilib>:"PID.vi"("output range"=cluster{"output high":dbl, "output low":dbl} {"output high"=1.0, "output low"=-1.0}, "PID gains"="Camera Tracking", "setpoint"=w309) -> ("output"=w307:dbl)  [unwired: 7 in, 1 out]
          n296 = global write "Driver Controller Global.vi" "Rumble Controller?"(FALSE ("Rumble Controller?")) -> ()
          n297 = Multiply(x=w306, y=w307) -> (x*y=w308:dbl)
        }
      }
    }
  }
  n298 = global write "Drive Train Global.vi" "Z Command"(w48) -> ()
  n299 = global write "Drive Train Global.vi" "X Command"(w46) -> ()
